vi "CS POLARIS BME DG.constructor.vi"(0 "name":string, 2 "data in":string, 5 "error in (no error)":errorcluster) -> (14 "i ref out":refnum<vi>, 16 "data out":string, 19 "error out":errorcluster)   [LabVIEW 2009, in "CS POLARIS BME DG.lvlib"]
doc: "This is the constructor of a class.\n\nLicense Agreement for this software:\n\nCopyright (C)\nGesellschaft für Schwerionenforschung, GSI\nPlanckstr. 1\n64291 Darmstadt\nGermany\n\nContact: D.Beck@gsi.de \n\nThis program is free software; you can redistribute it and/or modify it under the terms of the \nGNU General Public License as published by the Free Software Foundation; either version 2 of \nthe license, or (at your option) any later version.\n\nThis program is distributed in the hope that it will be useful, but WITHOUT ANY WARRANTY; \nwithout even the implied warranty of MERCHANTABILITY or FITNESS FOR A PARTICULAR PURPOSE. See the GNU General License for more details (http://www.gnu.org).\n\nGesellschaft für Schwerionenforschung, GSI\nPlanckstr. 1, 64291 Darmstadt, Germany\nFor all questions and ideas contact: M.Richter@gsi.de, H.Brand@gsi.de or D.Beck@gsi.de.\nLast update: 16-JUN-2004"
uses:
  CS POLARIS BME DG.lvlib
  CSApplicationBaseClasses/DeviceBase/DeviceBase.deviceState.ctl
  DG Classes/BME_DG_System/ChnlOutputModulo.ctl
  CSApplicationBaseClasses/DeviceBase/DeviceBase.myEventNames.ctl
  CSApplicationBaseClasses/DeviceBase/DeviceBase.lvlib
  CSCore/CSSystem/CSSystemLib/CSSystemLib.lvlib
  POLARIS BME DG.lvlib
  DG Classes/BME_DG_System/BME_DG_System.lvclass
  CSCore/BaseProcess/BaseProcess.lvlib
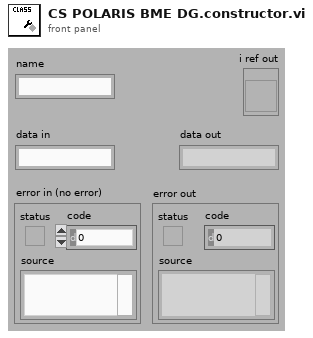
[diagram p1: front panel]
types:
  T1 = typedef "POLARIS BME DG.lvlib/ChnlOutputModulo.ctl" = cluster{"ChnlName":string, "TriggerModulo":u32}
  T2 = enum16{"SetAttribute", "GetAttribute", "CreateAttribute", "DestroyAttribute", "DestroyAllAtributes"}
  T3 = typedef "DeviceBase.lvlib/DeviceBase.deviceState.ctl" = i16
  T4 = typedef "DeviceBase.lvlib/DeviceBase.myEventNames.ctl" = enum16{"lvmsg://Initialize", "lvmsg://Close", "lvmsg://Configure", "lvmsg://Reset", "lvmsg://IDQuery"}
  T5 = typedef "BaseProcess.lvlib/BaseProcess.i attribute.ctl" = cluster{"EventStatus":string, "EventError":i32, "PresetEvtWatchD":i32, "PresetPdcWatchD":i32, "EventTimeout":i32, "PeriodicInterval":i32, "Interface":string[], "Address":string[], "Special":string[], "PeriodicError":i32, "PeriodicStatus":string, "SuperProc":string, "Descriptors":T6[], "CaseRef":refnum<vi>, "PdcRef":refnum<vi>, "Thread Ref":refnum<vi>, "eventErrorID":i32, "eventStatusID":i32, "periodicErrorID":i32, "periodicStatusID":i32, "pdcCtrID":i32}
  T6 = typedef "BaseProcess.lvlib/BaseProcess.descriptor definition.ctl" = cluster{"selector":string, "descriptor":T7}
  T7 = typedef "BaseProcess.lvlib/BaseProcess.descriptor string definition.ctl" = string
  T8 = typedef "CS POLARIS BME DG.lvlib/CS POLARIS BME DG.i attribute.ctl" = cluster{"Numeric":dbl, "DG_System":refnum<queue>, "UpdateTasks":refnum<queue>}
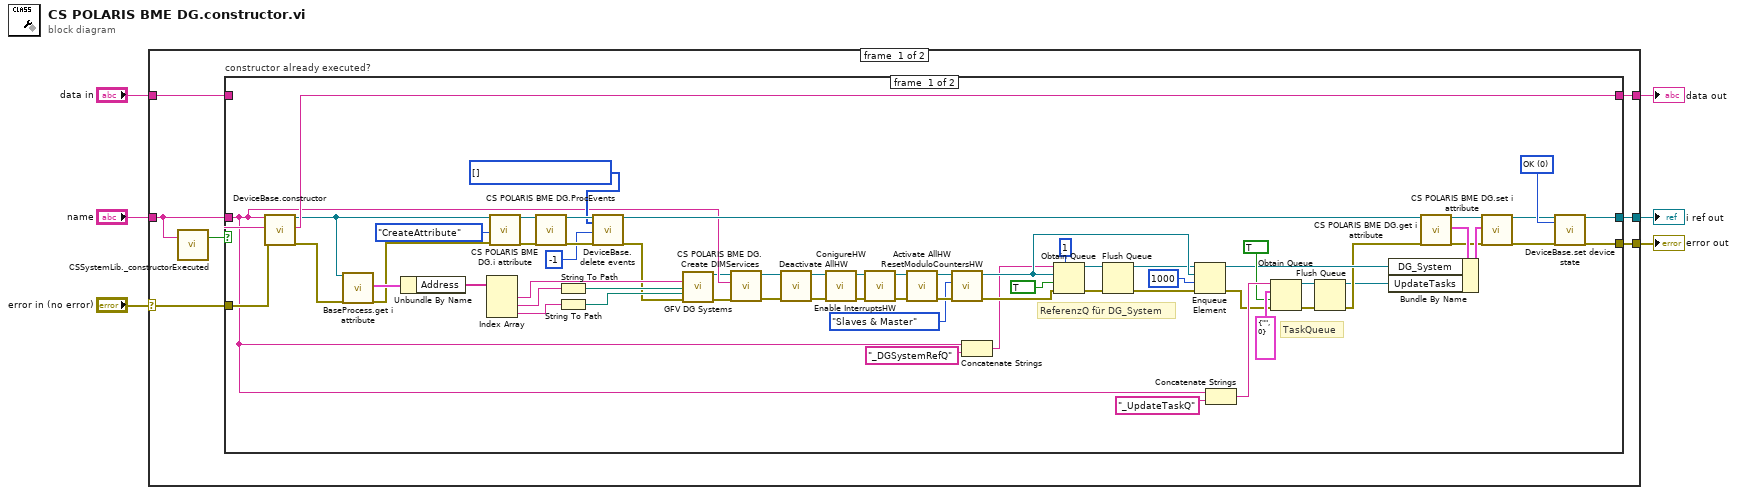
[diagram p0: block diagram]
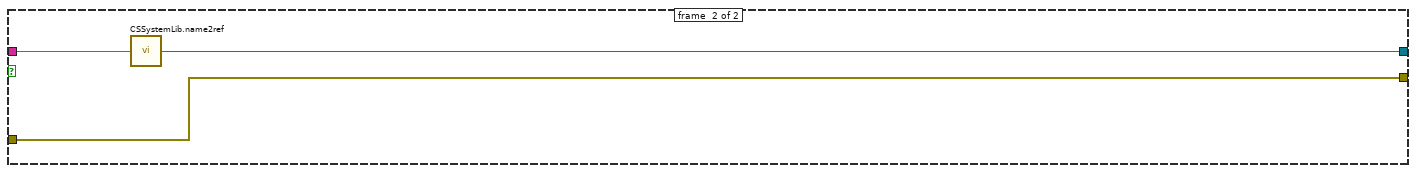
[diagram p2: hidden frame]
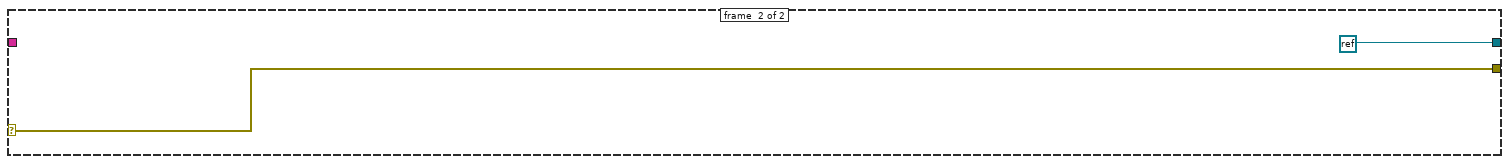
[diagram p3: hidden frame]
diagram:
  n1 = case shown="No Error" "error in (no error)" {
    selector: "error in (no error)" -> [w11 w83]
    tunnel: "name" -> [w10 _]
    tunnel: [w13 refnum<k0> refnum ("Not a Refnum Constant")] -> w5
    tunnel: [w12 w83] -> w4
    tunnel: "data in" -> [w8 _]
    tunnel: [w7 _] -> w1
    frame #0 {
      n2 = call "CSSystemLib._constructorExecuted.vi"("name"=w10) -> ("constructor executed?"=w9:bool)  [unwired: 18 in]
      n3 = case "constructor already executed?" shown="False" w9 {
        tunnel: w10 -> [w28 w82]
        tunnel: [w33 w81] -> w13
        tunnel: [w31 w80] -> w12
        tunnel: w11 -> [w76 w80]
        tunnel: w8 -> [w75 _]
        tunnel: [w70 _] -> w7
        frame #0 {
          w54 = T3 0 items=["ERROR"=-1, "OK"=0, "NOT_OK"=1] ("deviceState")
          w72 = T4[] [] items=["lvmsg://Initialize", "lvmsg://Close", "lvmsg://Configure", "lvmsg://Reset", "lvmsg://IDQuery"] ("events")
          # "ReferenzQ für DG_System"
          # "TaskQueue"
          n4 = call "DeviceBase.constructor.vi"("name"=w28, "data in"=w75, "error in (no error)"=w76) -> ("i ref out"=w26:refnum<vi>, "data out"=w70:string, "error out"=w25:errorcluster)  [unwired: 14 in]
          n5 = call "BaseProcess.get i attribute.vi"("i ref in"=w26, "error in (no error)"=w25) -> ("i attribute"=w24:T5, "error out"=w22:errorcluster)  [unwired: 15 in, 1 out]
          n6 = Unbundle By Name(w24) -> ("Address"=w23:string[])
          n7 = Index Array(array=w23) -> (element #1=w18:string, element #2=w17:string, element #3=w16:string)  [unwired: 3 in]
          n8 = call "CS POLARIS BME DG.i attribute.vi"("VI Refnum"=w26, "Action"=T2."CreateAttribute", "error in (no error)"=w22) -> ("VI Refnum out"=w78:refnum<vi>, "error out"=w77:errorcluster)  [unwired: 14 in, 1 out]
          n9 = call "CS POLARIS BME DG.ProcEvents.vi"("i ref in"=w78, "error in (no error)"=w77) -> ("i ref out"=w74:refnum<vi>, "error out"=w73:errorcluster)  [unwired: 16 in]
          n10 = String To Path(string=w17) -> (path=w20:path)
          n11 = String To Path(string=w16) -> (path=w19:path)
          n12 = call "DeviceBase.delete events.vi"("i ref in"=w74, "events"=w72, "ms timeout (10000)"=-1, "error in (no error)"=w73) -> ("i ref out"=w61:refnum<vi>, "error out"=w15:errorcluster)  [unwired: 13 in, 1 out]
          n13 = call "GFV DG Systems.vi"("SystemlName"=w18, "Config File"=w20, "Dir Calibration files"=w19, "error in"=w15) -> ("BME_DG_System out"=w21:refnum<class "BME_DG_System.lvclass">, "error out"=w14:errorcluster)  [unwired: 6 in, 4 out]
          n14 = call "CS POLARIS BME DG.Create DIMServices.vi"("error in (no error)"=w14, "objname"=w28, "BME_DG_System in"=w21) -> ("error out"=w29:errorcluster, "BME_DG_System out"=w30:refnum<class "BME_DG_System.lvclass">)  [unwired: 7 in]
          n15 = call "Deactivate AllHW.vi"("error in (no error)"=w29, "BME_DG_System in"=w30) -> ("error out"=w52:errorcluster, "BME_DG_System out"=w53:refnum<class "BME_DG_System.lvclass">)  [unwired: 8 in]
          n16 = call "ConigureHW.vi"("error in (no error)"=w52, "BME_DG_System in"=w53) -> ("error out"=w50:errorcluster, "BME_DG_System out"=w51:refnum<class "BME_DG_System.lvclass">)  [unwired: 8 in]
          n17 = call "Enable InterruptsHW.vi"("error in (no error)"=w50, "BME_DG_System in"=w51) -> ("error out"=w48:errorcluster, "BME_DG_System out"=w49:refnum<class "BME_DG_System.lvclass">)  [unwired: 8 in]
          n18 = call "Activate AllHW.vi"("error in (no error)"=w48, "BME_DG_System in"=w49) -> ("error out"=w46:errorcluster, "BME_DG_System out"=w47:refnum<class "BME_DG_System.lvclass">)  [unwired: 8 in]
          n19 = call "ResetModuloCountersHW.vi"("error in (no error)"=w46, "Enum"=enum16{"Slaves only", "Slaves & Master"}."Slaves & Master", "BME_DG_System in"=w47) -> ("error out"=w44:errorcluster, "BME_DG_System out"=w43:refnum<class "BME_DG_System.lvclass">)  [unwired: 7 in]
          n20 = Concatenate Strings(w28, "_DGSystemRefQ" ("string")) -> (w27:string)
          n21 = Obtain Queue(max queue size (-1, unlimited)=1, name (unnamed)=w27, element data type=w43, create if not found? (T)=TRUE, error in (no error)=w44) -> (queue out=w41:refnum<queue>, error out=w42:errorcluster)  [unwired: 1 out]
          n22 = Flush Queue(queue=w41, error in (no error)=w42) -> (queue out=w39:refnum<queue>, error out=w40:errorcluster)  [unwired: 1 out]
          n23 = Enqueue Element(queue=w39, element=w43, timeout in ms (-1)=1000, error in (no error)=w40) -> (queue out=w57:refnum<queue>, error out=w56:errorcluster)  [unwired: 1 out]
          n24 = Concatenate Strings(w28, "_UpdateTaskQ" ("string")) -> (w65:string)
          n25 = Obtain Queue(name (unnamed)=w65, element data type=T1 {"ChnlName"="", "TriggerModulo"=0} ("UpdateChnlTask"), create if not found? (T)=TRUE, error in (no error)=w56) -> (queue out=w36:refnum<queue>, error out=w38:errorcluster)  [unwired: 1 in, 1 out]
          n26 = Flush Queue(queue=w36, error in (no error)=w38) -> (queue out=w35:refnum<queue>, error out=w37:errorcluster)  [unwired: 1 out]
          n27 = call "CS POLARIS BME DG.get i attribute.vi"("i ref in"=w61, "error in (no error)"=w37) -> ("i ref out"=w62:refnum<vi>, "i attribute"=w60:T8, "error out"=w58:errorcluster)  [unwired: 15 in]
          n28 = Bundle By Name(cluster=w60, "DG_System"=w57, "UpdateTasks"=w35) -> (w59:T8)
          n29 = call "CS POLARIS BME DG.set i attribute.vi"("i ref in"=w62, "i attribute"=w59, "error in (no error)"=w58) -> ("i ref out"=w34:refnum<vi>, "error out"=w32:errorcluster)  [unwired: 15 in]
          n30 = call "DeviceBase.set device state.vi"("i ref in"=w34, "deviceState"=w54, "error in (no error)"=w32) -> ("i ref out"=w33:refnum<vi>, "error out"=w31:errorcluster)  [unwired: 14 in, 1 out]
        }
        frame #1 {
          n31 = call "CSSystemLib.name2ref.vi"("name"=w82) -> ("obj refnum"=w81:refnum<vi>)
        }
      }
    }
    frame #1 {
    }
  }
  "i ref out" <- w5
  "error out" <- w4
  "data out" <- w1
